vi "load config.vi"(8 "error in (no error)":errorcluster, 10 "TABLE":string="power_environment_monitoring", 11 "VI引用句柄":refnum<vi>) -> (0 "error out":errorcluster)   [LabVIEW 2016]
uses:
  <userlib>/_LVST/sqlite_api/Core/Select/SQLite_Select Str.vi
panel:
  out "数组":T1(array[cluster])
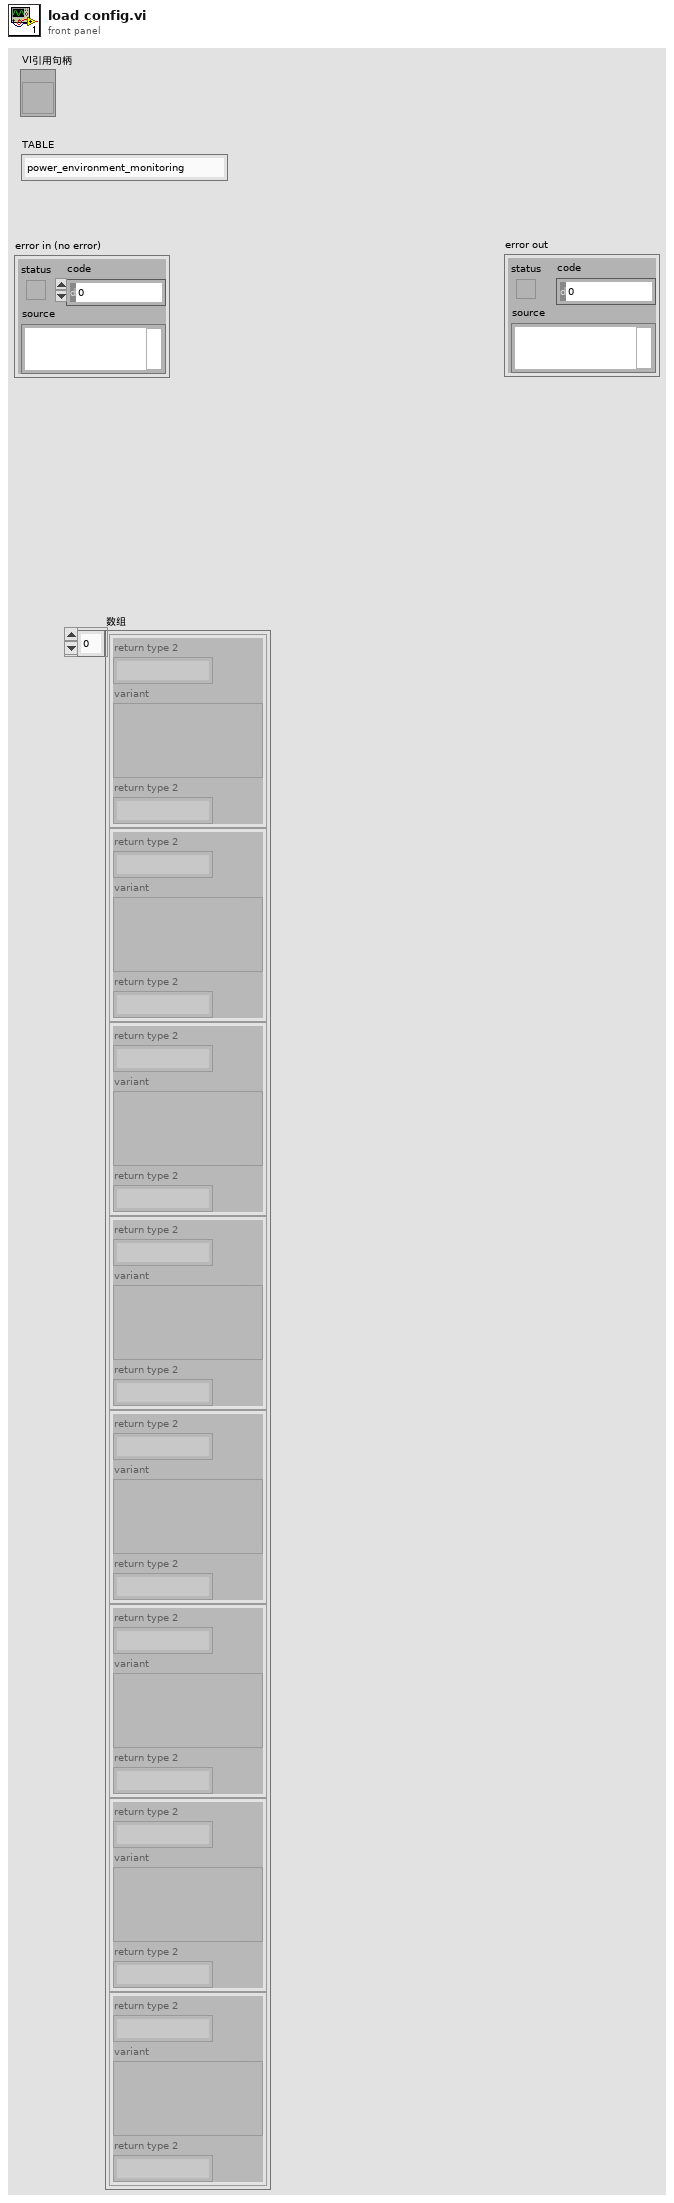
[diagram p1: front panel]
types:
  T1 = cluster{"return type 2":string, "variant":variant, "return type 2":string}[]
  T2 = cluster{"return type 2":string, variant, "return type 2":string}
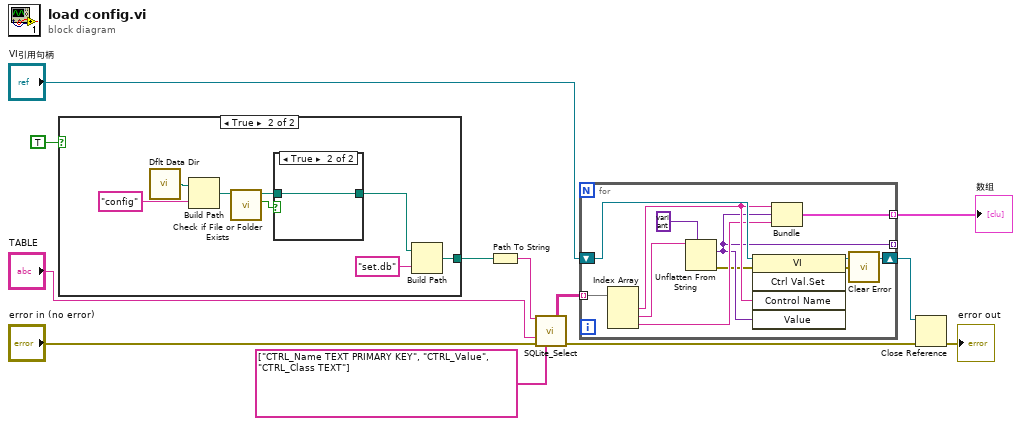
[diagram p0: block diagram]
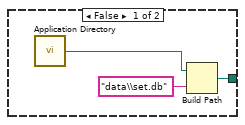
[diagram p2: hidden frame]
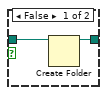
[diagram p3: hidden frame]
diagram:
  n1 = case shown="True" TRUE {
    tunnel: [w13 w16] -> w1
    frame False {
      n2 = call <vilib>:"Application Directory.vi"() -> ("Application Directory"=w15:path)
      n3 = Build Path(base path=w15, name or relative path="data\\set.db" ("名称或相对路径")) -> (appended path=w13:path)
    }
    frame True {
      n4 = call <vilib>:"Dflt Data Dir.vi"() -> ("App:Default Data Directory"=w23:path)
      n5 = Build Path(base path=w23, name or relative path="config" ("名称或相对路径")) -> (appended path=w21:path)
      n6 = call <vilib>:"Check if File or Folder Exists.vi"("path"=w21) -> ("file or folder exists?"=w20:bool, "dup path"=w19:path)  [unwired: 8 in, 1 out]
      n7 = case shown="True" w20 {
        tunnel: w19 -> [w25 w26]
        tunnel: [w24 w26] -> w18
        frame False {
          n8 = Create Folder(path (use dialog)=w25) -> (created path=w24:path)  [unwired: 2 in, 2 out]
        }
        frame True {
        }
      }
      n9 = Build Path(base path=w18, name or relative path="set.db" ("名称或相对路径")) -> (appended path=w16:path)
    }
  }
  n10 = Path To String(path=w1) -> (string=w12:string)
  n11 = call-poly <userlib>:"SQLite_Select.vi"("DB Path"=w12, "Table Name"="TABLE", "error in (no error)"="error in (no error)", "Columns"=string[] ["CTRL_Name TEXT PRIMARY KEY", "CTRL_Value", "CTRL_Class TEXT"] ("Column")) -> ("Results"=w6:string[][], "error out"=w9:errorcluster)  [unwired: 8 in, 2 out]
  n12 = for {
    tunnel: w6 -> [w37] mode=indexing
    shift-right: [w34] -> w10
    shift-left: "VI引用句柄" -> [w36]
    tunnel: [w28] -> _ mode=indexing
    tunnel: [w31] -> w7 mode=indexing
    n13 = Index Array(array=w37) -> (element #1=w33:string, element #2=w30:string, element #3=w32:string)  [unwired: 3 in]
    n14 = Unflatten From String(type=variant, binary string=w30) -> (value=w28:variant, error out=w27:errorcluster)  [unwired: 3 in, 1 out]
    n15 = invoke class="VI" method="Ctrl Val.Set"(reference=w36, error in=w27, "Control Name"=w33, "Value"=w28) -> (reference out=w34:refnum<vi>, error out=w35:errorcluster)  [unwired: 1 in, 3 out]
    n16 = Bundle("return type 2"=w33, w28, "return type 2"=w32) -> (w31:T2)  [unwired: 1 in]
    n17 = call <userlib>:"Clear Error.vi"("error in (no error)"=w35) -> ()  [unwired: 4 in, 1 out]
  }
  "数组" <- w7
  n18 = Close Reference(reference=w10, error in (no error)=w9) -> (error out=→"error out":errorcluster)
